vi "CriticalComponents.vi"() -> ()   [LabVIEW 2014]
uses:
  <vilib>/Instr/_visa.llb/VISA Configure Serial Port (Instr).vi
  <vilib>/FieldPoint/Polymorphic Read.llb/FP Read (Float -IO).vi
  <vilib>/FieldPoint/Polymorphic Write.llb/FP Write (Float -IO).vi
  <vilib>/FieldPoint/Polymorphic Write.llb/FP Write (Boolean -IO).vi
  GlobalVariables.vi
panel:
  in  "Tab Control":enum32{"Main", "Email/Text", "Errors", "Misc."}(tab)
  in  "Detector":bool
  in  "Shield":bool
  in  "SC":bool
  out "Pos. Current Readout 2":dbl=1e-05 format="%#.2g"
  out "Neg. Current Readout 2":dbl=1e-05 format="%#.2g"
  out "+ Plate (kV)":dbl
  out "- Plate (kV)":dbl
  out "Current status":bool
  out "Current status 2":bool
  in  "WF Set Point":dbl=0.01 min=0.0 max=10.0 step=0.01 format="%#_3g"
  in  "Auto-Set WF":bool
  in  "Master Voltage control":dbl caption="Set both plate voltages" min=0.0 max=10.0 step=0.01 format="%#_3g"
  in  "stop":bool
  out "Mag. Field (T)":string
  out "Spec Vac":bool
  in  "Spec":bool=TRUE
  out "SC Vac":bool
  in  "SC":bool=TRUE
  out "BL Vac":bool
  in  "BL":bool=TRUE
  in  "Spec turbo\nvalve ctrl":bool
  out "Boolean 9":bool
  in  "Boolean 15":bool
  out "Boolean 8":bool
  in  "BL Ctrl":bool
  out "Boolean 11":bool
  out "Boolean 12":bool
  out "Boolean 13":bool
  in  "Alpha Ctrl":bool
  out "Boolean 10":bool
  in  "Fil on/ 21":bool
  in  "Fil off/ 20":bool
  out "Scat. Chamber":string
  out "Scatt TC (Torr)":string
  in  "BL IG Fil on":bool
  in  "BL IG Fil off":bool
  in  "BL Degas on":bool
  out "Beamline":string
  out "Beamline TC1 (Torr) 2":string
  out "Spectrograph\nVacuum":string
  out "Spectrograph 2 (High Vac)":string
  in  "phone number":string
  in  "Carrier":enum16{"T-Mobile", "AT&T", "Verizon", "Sprint"}(ring)
  in  "On Call":bool
  in  "Write":bool
  in  "Text Body":string
  in  "Text Subject":string="Vacuum Status!"
  in  "Tyler":bool=TRUE
  in  "Michael":bool=TRUE
  in  "Karen":bool=TRUE
  in  "sendbutton":bool
  in  "Tyler Email":bool=TRUE
  in  "Michael Email":bool=TRUE
  in  "Karen Email":bool=TRUE
  in  "Email Message":string caption="Message"
  in  "Email Subject":string caption="Subject"
  in  "Email Send":bool
  out "WF Pos Current":errorcluster caption="error out"
  out "WF Pos Voltage":errorcluster caption="error out"
  out "Spec Ctrl":errorcluster caption="error out"
  out "Spec Close":errorcluster caption="error out"
  out "Spec Open":errorcluster caption="error out"
  out "BL Ctrl 2":errorcluster caption="error out"
  out "BL Close":errorcluster caption="error out"
  out "BL Open":errorcluster caption="error out"
  out "Alpha Ctrl 2":errorcluster caption="error out"
  out "Alpha Close":errorcluster caption="error out"
  out "Alpha Open":errorcluster caption="error out"
  out "WF Neg Current":errorcluster caption="error out"
  out "WF Neg Voltage":errorcluster caption="error out"
  out "BL Cup Error Status":errorcluster caption="error out"
  in  "WF, Comm 34, F":refnum<visa-resource-name>="COM34"
  in  "Spect Vac, Comm 35, A":refnum<visa-resource-name>="COM35"
  in  "BL Vac, Comm 32, G":refnum<visa-resource-name>="COM32"
  out "WF Volt Error":errorcluster caption="error out"
  out "WF Volt Error 2":errorcluster caption="error out"
  out "6600 V1":dbl
  out "6600 V3":dbl
  out "4500 TC1":dbl
  out "4500 IG":dbl
  out "4500 TC2":dbl
  out "4500 TC1 2":dbl
  out "Beamline TC1 (Torr)":string
  out "Spec 2 (high vac) hidden":dbl
  out "x-y":i32
  in  "BL Degas off":bool
  out "Boolean 14":bool
  out "?":bool=TRUE
  out "Vac Indicator":bool=TRUE
  in  "GFM":bool
  in  "Vanilla IC":bool=TRUE
  in  "smtp server":string="smtp.gmail.com"
  in  "show errors 2":bool
  in  "Teslameter Port 5":refnum<visa-resource-name>="COM34"
  # "Overrrides"
  # "Select who receives the email. Green=recieves, Grey =doesn't receive."
  # "Select who receives the text. Green = recieves. Grey = doesn't recieve."
  # "Beam Line IG"
  # "Variable for WF Auto Set"
  # "Scattering Chamber IC"
  # "Not currently working"
  # "For sending emails"
  # "Indicators and Controls not in use."
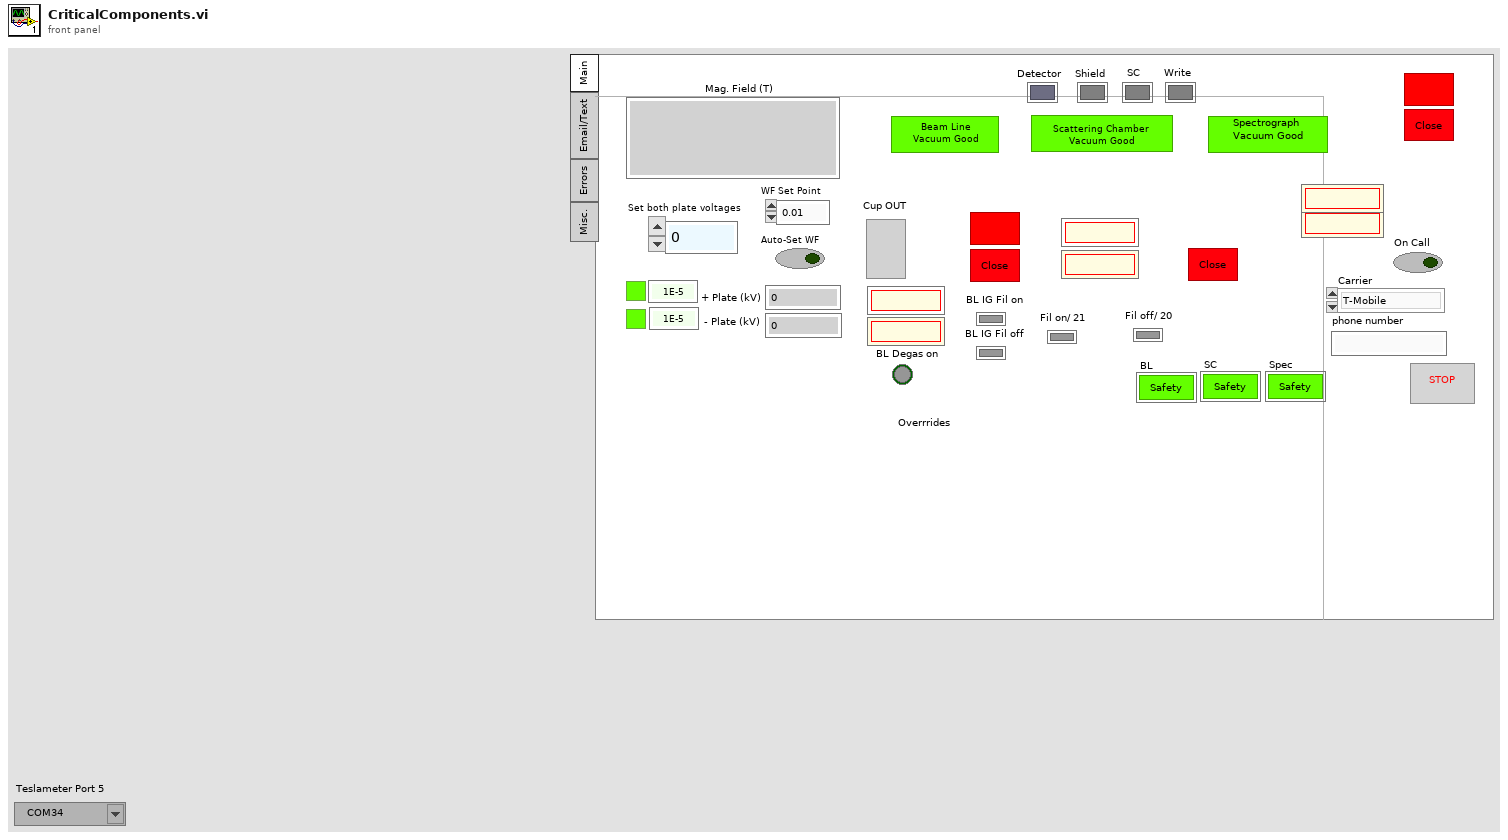
[diagram p1: front panel]
types:
  T1 = enum32{"Invalid", "Standard", "Closed", "Hidden", "Minimized", "Maximized"}
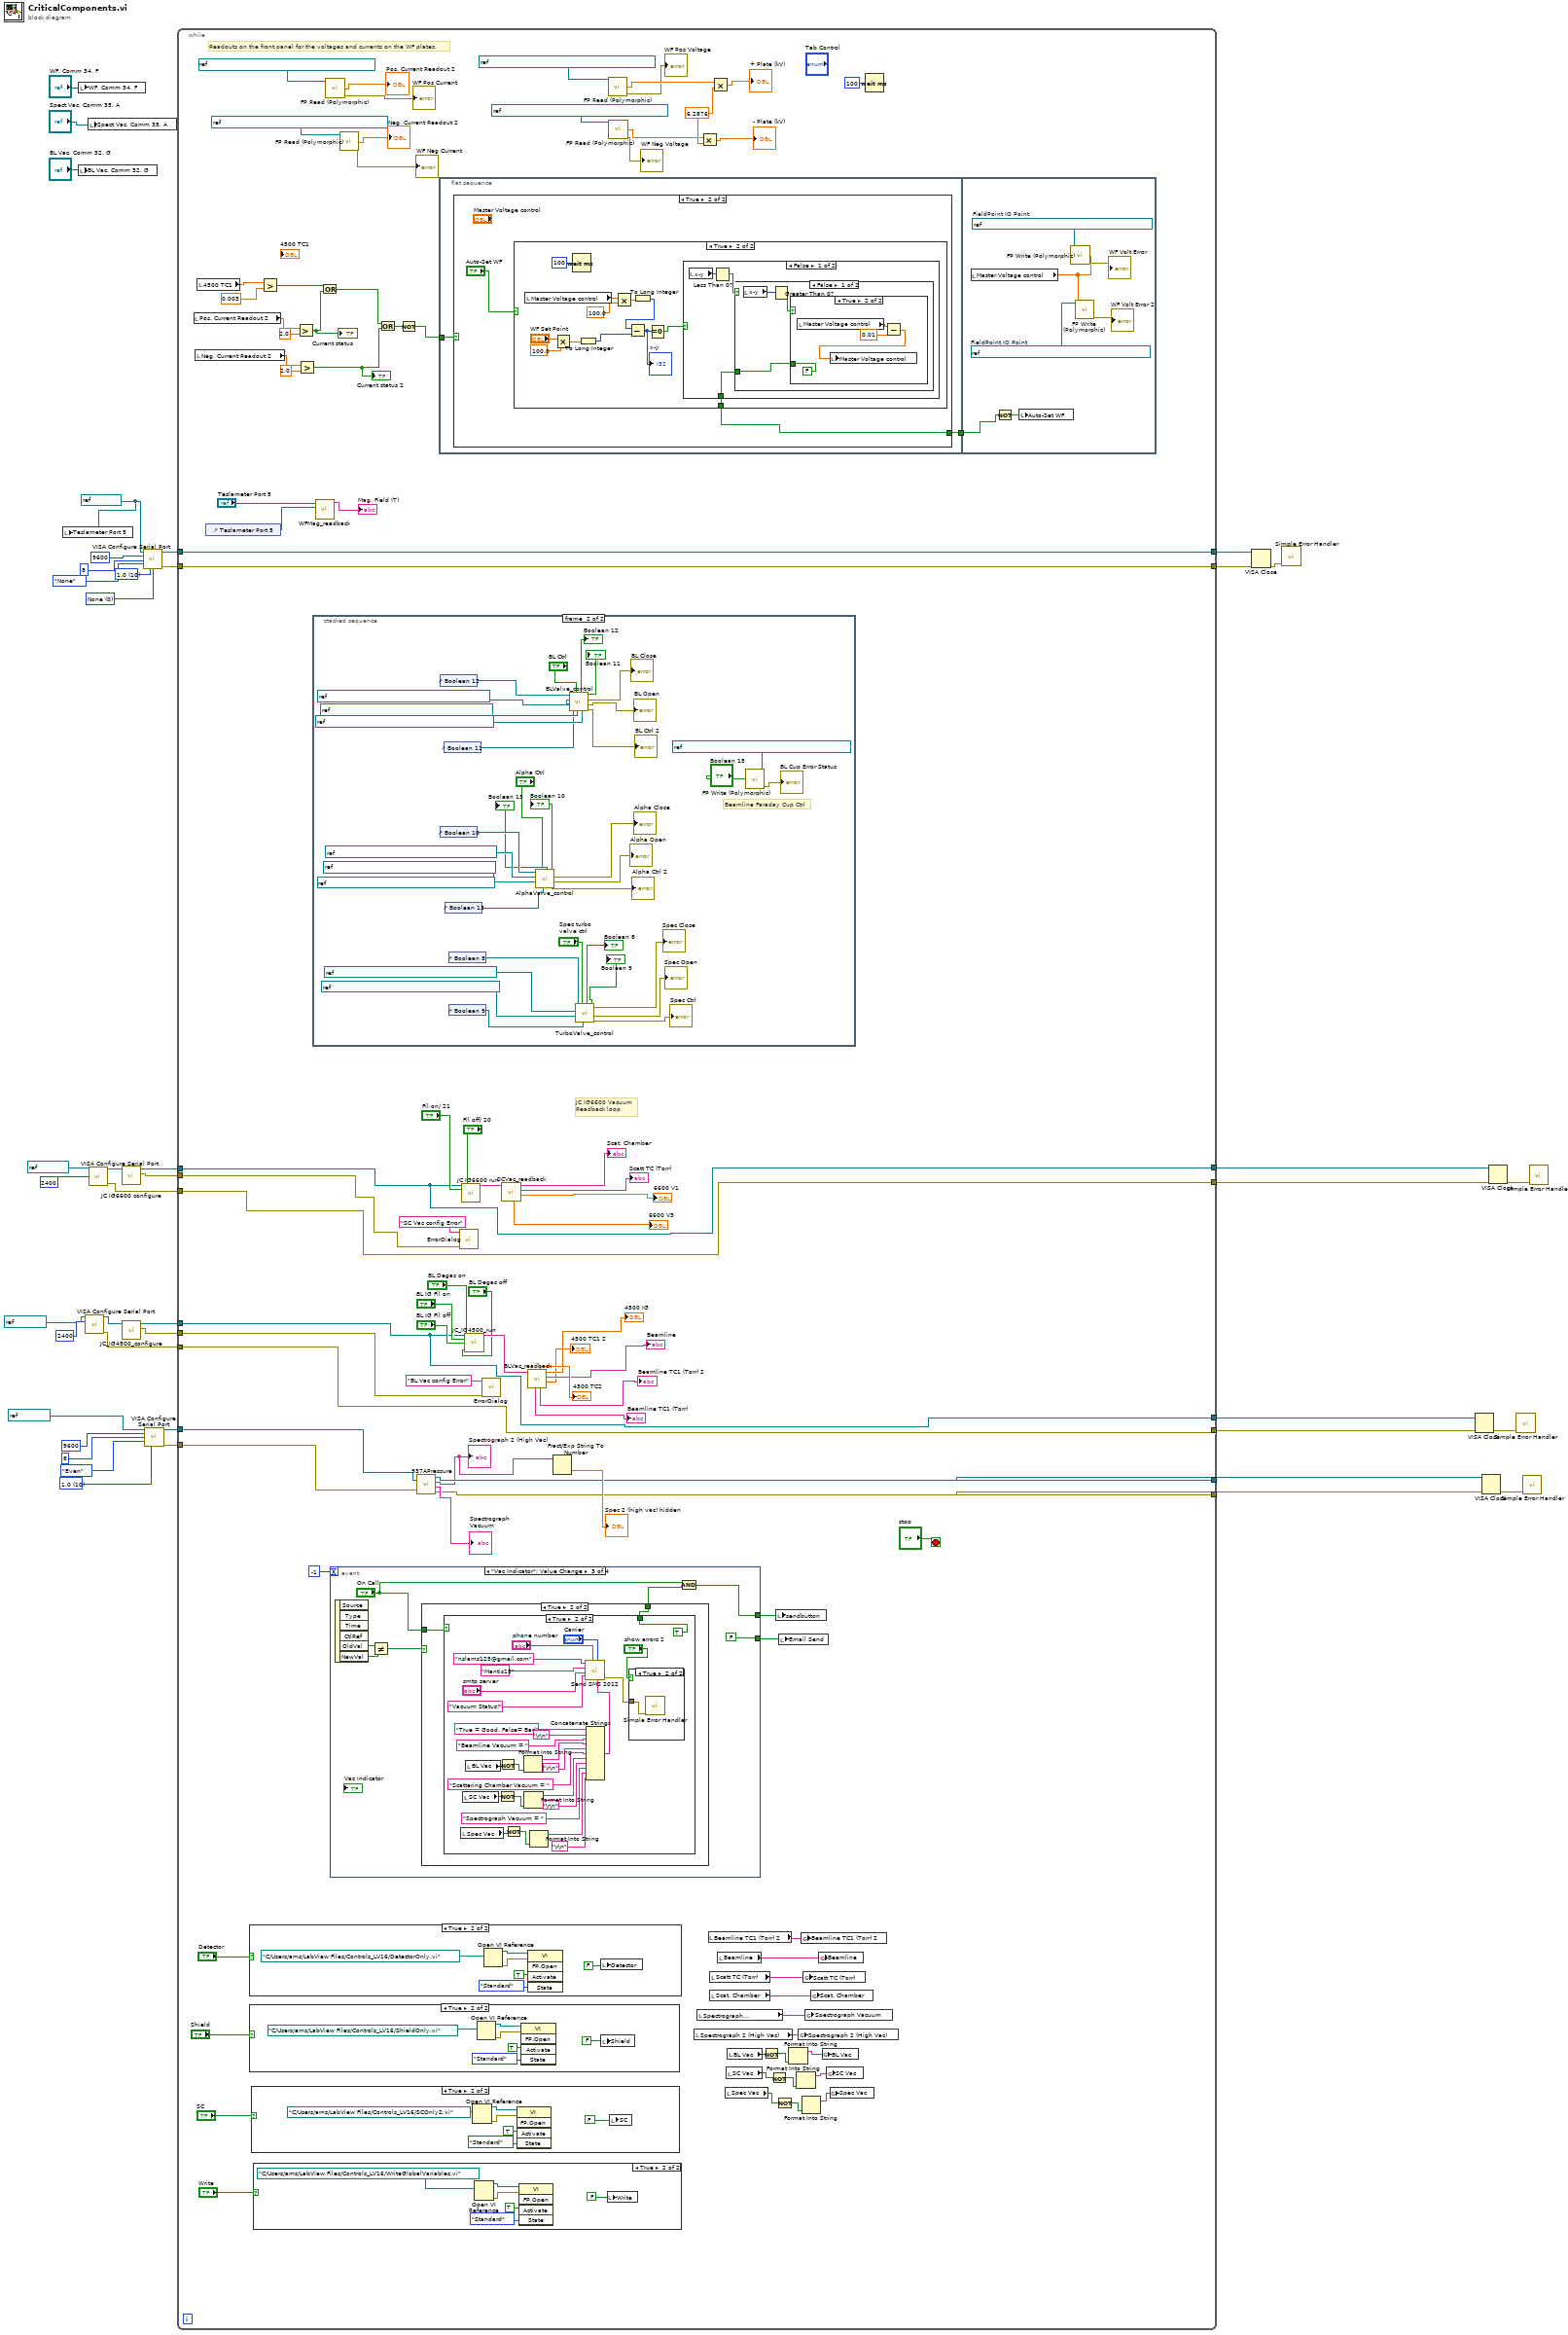
[diagram p0: block diagram]
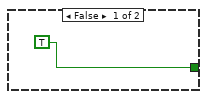
[diagram p2: hidden frame]
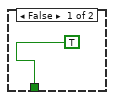
[diagram p3: hidden frame]
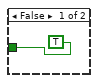
[diagram p4: hidden frame]
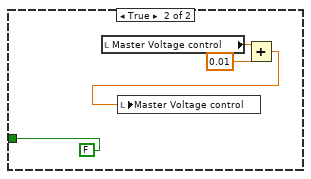
[diagram p5: hidden frame]
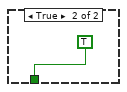
[diagram p6: hidden frame]
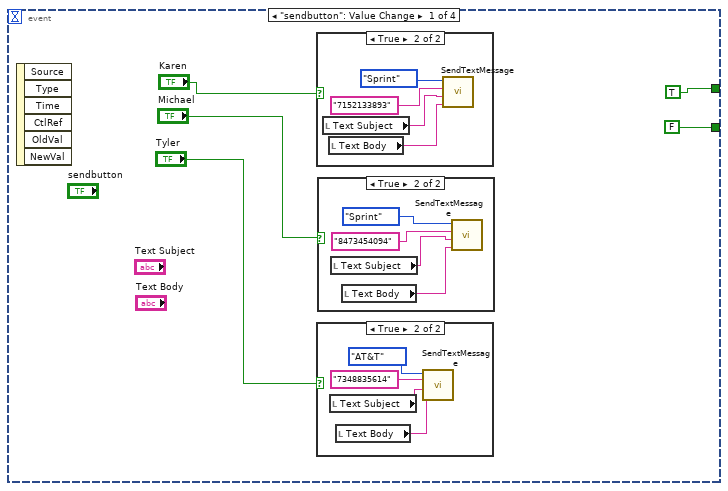
[diagram p11: hidden frame]
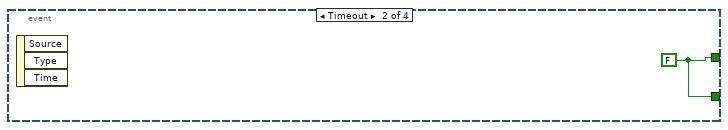
[diagram p15: hidden frame]
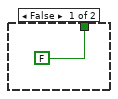
[diagram p16: hidden frame]
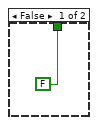
[diagram p17: hidden frame]
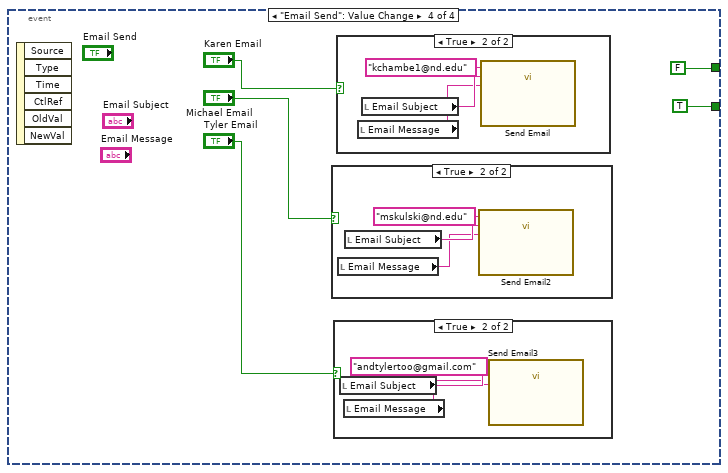
[diagram p19: hidden frame]
diagram:
  w7 = u16 10 items=["1.0"=10, "1.5"=15, "2.0"=20] ("stop bits (10: 1 bit)")
  w34 = refnum<visa-resource-name> "COM34" ("VISA resource name")
  w35 = u16 0 items=["None", "XON/XOFF", "RTS/CTS", "XON/XOFF & RTS/CTS", "DTR/DSR", "XON/XOFF & DTR/DSR"] ("flow control (0:none)")
  w36 = u16 10 items=["1.0"=10, "1.5"=15, "2.0"=20] ("stop bits (10: 1 bit)")
  n1 = local write "Teslameter Port 5"(w34) -> ()
  n2 = local write "BL Vac, Comm 32, G"("BL Vac, Comm 32, G") -> ()
  n3 = local write "WF, Comm 34, F"("WF, Comm 34, F") -> ()
  n4 = call-poly "VISA Configure Serial Port"("VISA resource name"=refnum<visa-resource-name> "COM32" ("VISA IN (Default COM9)"), "baud rate (9600)"=u32 2400) -> ("VISA resource name out"=w13:refnum<visa-resource-name>, "error out"=w8:errorcluster)  [unwired: 12 in]
  n5 = local write "Spect Vac, Comm 35, A"("Spect Vac, Comm 35, A") -> ()
  n6 = call-poly "VISA Configure Serial Port"("VISA resource name"=refnum<visa-resource-name> "COM31" ("VISA IN (Default COM4)"), "baud rate (9600)"=u32 2400) -> ("VISA resource name out"=w19:refnum<visa-resource-name>, "error out"=w15:errorcluster)  [unwired: 12 in]
  n7 = call "JC IG6600 configure.vi"("VISA IN (Default COM4)"=w19) -> ("Error"=w14:errorcluster, "VISA resource name out"=w16:refnum<visa-resource-name>)  [unwired: 9 in]
  n8 = call "JC_IG4500_configure.vi"("VISA IN (Default COM9)"=w13) -> ("Error"=w9:errorcluster, "VISA resource name out"=w10:refnum<visa-resource-name>)  [unwired: 9 in]
  n9 = call-poly "VISA Configure Serial Port"("VISA resource name"=w34, "baud rate (9600)"=u32 9600, "data bits (8)"=u16 8, "parity (0:none)"=enum16{"None", "Odd", "Even", "Mark", "Space"}."None", "stop bits (10: 1 bit)"=w36, "flow control (0:none)"=w35) -> ("VISA resource name out"=w33:refnum<visa-resource-name>, "error out"=w32:errorcluster)  [unwired: 8 in]
  n10 = call-poly "VISA Configure Serial Port"("VISA resource name"=refnum<visa-resource-name> "COM35", "baud rate (9600)"=u32 9600, "data bits (8)"=u16 8, "parity (0:none)"=enum16{"None", "Odd", "Even", "Mark", "Space"}."Even", "stop bits (10: 1 bit)"=w7) -> ("VISA resource name out"=w2:refnum<visa-resource-name>, "error out"=w1:errorcluster)  [unwired: 9 in]
  n11 = while {
    tunnel: w33 -> [w102]
    tunnel: w32 -> [w101]
    tunnel: [w102] -> w30
    tunnel: [w101] -> w31
    tunnel: [w50] -> w26
    tunnel: [w47] -> w28
    tunnel: [w56] -> w24
    tunnel: [w55] -> w23
    tunnel: [w51] -> w21
    tunnel: [w53] -> w20
    tunnel: w16 -> [w56]
    tunnel: w15 -> [w55]
    tunnel: w14 -> [w54]
    tunnel: w10 -> [w53]
    tunnel: w9 -> [w52]
    tunnel: w8 -> [w51]
    tunnel: w2 -> [w46]
    tunnel: w1 -> [w45]
    stop <- "stop" stop-if-true
    w125 = 6.2876
    # "JC IG6600 Vacuum \nReadback loop"
    # "Readouts on the front panel for the voltages and currents on the WF plates."
    n12 = local read "Pos. Current Readout 2"() -> (w116:dbl)
    n13 = local read "Neg. Current Readout 2"() -> (w112:dbl)
    n14 = local read "4500 TC1"() -> (w118:dbl)
    n15 = control-ref of="Teslameter Port 5"() -> (w105:refnum<vi>)
    n16 = case shown="True" "Detector" {
      frame False {
      }
      frame True {
        n17 = Open VI Reference(vi path=path "C:/Users/ams/LabView Files/Controls_LV16/DetectorOnly.vi") -> (vi reference=w192:refnum<vi>, error out=w197:errorcluster)  [unwired: 5 in]
        n18 = invoke class="VI" method="FP.Open"(reference=w192, error in=w197, "Activate"=TRUE ("Activate?"), "State"=T1."Standard") -> ()  [unwired: 1 in, 5 out]
        n19 = local write "Detector"(FALSE) -> ()
      }
    }
    n20 = case shown="True" "Shield" {
      frame False {
      }
      frame True {
        n21 = Open VI Reference(vi path=path "C:/Users/ams/LabView Files/Controls_LV16/ShieldOnly.vi") -> (vi reference=w186:refnum<vi>, error out=w191:errorcluster)  [unwired: 5 in]
        n22 = invoke class="VI" method="FP.Open"(reference=w186, error in=w191, "Activate"=TRUE ("Activate?"), "State"=T1."Standard") -> ()  [unwired: 1 in, 5 out]
        n23 = local write "Shield"(FALSE ("Boolean 2")) -> ()
      }
    }
    n24 = case shown="True" "SC" {
      frame False {
      }
      frame True {
        n25 = Open VI Reference(vi path=path "C:/Users/ams/LabView Files/Controls_LV16/SCOnly2.vi") -> (vi reference=w180:refnum<vi>, error out=w185:errorcluster)  [unwired: 5 in]
        n26 = invoke class="VI" method="FP.Open"(reference=w180, error in=w185, "Activate"=TRUE ("Activate?"), "State"=T1."Standard") -> ()  [unwired: 1 in, 5 out]
        n27 = local write "SC"(FALSE ("Boolean 3")) -> ()
      }
    }
    n28 = case shown="True" "Write" {
      frame False {
      }
      frame True {
        n29 = Open VI Reference(vi path=path "C:/Users/ams/LabView Files/Controls_LV16/WriteGlobalVariables.vi") -> (vi reference=w174:refnum<vi>, error out=w179:errorcluster)  [unwired: 5 in]
        n30 = invoke class="VI" method="FP.Open"(reference=w174, error in=w179, "Activate"=TRUE ("Activate?"), "State"=T1."Standard") -> ()  [unwired: 1 in, 5 out]
        n31 = local write "Write"(FALSE ("Boolean 3")) -> ()
      }
    }
    n32 = Greater?(x=w118, y=0.003) -> (0:w114:bool)
    n33 = Greater?(x=w116, y=2.0) -> (0:w113:bool)
    "Current status" <- w113
    n34 = Greater?(x=w112, y=2.0) -> (0:w108:bool)
    "Current status 2" <- w108
    n35 = stacked-sequence {
      frame #0 {
        # "Spec."
        # "SC"
        # "BL"
        n36 = case shown="True" "Spec" {
          frame False {
          }
          frame True {
            n37 = local read "Spec 2 (high vac) hidden"() -> (w284:dbl)
            n38 = Equal?(x=w284, y=0.0) -> (x = y?=w282:bool)
            n39 = Greater?(x=w284, y=0.0001) -> (0:w281:bool)
            n40 = Or(x=w282, y=w281) -> (x .or. y?=w278:bool)
            "Spec Vac" <- w278
            n41 = case shown="False" "Vanilla IC" {
              tunnel: w278 -> [w291 w294]
              frame False {
                n42 = case shown="True" w291 {
                  selector: w291 -> [_ w293]
                  frame False {
                  }
                  frame True {
                    # "Spec in Safety + Vanilla IC = \nonly Turbo will close."
                    n43 = Not(x=w293) -> (.not. x?=w292:bool)
                    n44 = local write "Spec turbo\nvalve ctrl"(w292) -> ()
                  }
                }
              }
              frame True {
                # "Spec in Saftey + NO Vanilla IC = \nTurbo and Alpha will close."
                n45 = case shown="False" w294 {
                  selector: w294 -> [_ w296]
                  frame False {
                  }
                  frame True {
                    n46 = Not(x=w296) -> (.not. x?=w295:bool)
                    n47 = local write "Alpha Ctrl"(w295) -> ()
                    n48 = local write "Spec turbo\nvalve ctrl"(w295) -> ()
                  }
                }
              }
            }
            n49 = case shown="False" "GFM" {
              tunnel: w278 -> [w287 w288]
              frame False {
                # "Spec in Safety + GFM =\nTurbo will close."
                n50 = Not(x=w287) -> (.not. x?=w286:bool)
                n51 = local write "Spec turbo\nvalve ctrl"(w286) -> ()
              }
              frame True {
                # "Spec in Safety + NON GFM=\nTurbo and Alpha will close."
                n52 = case shown="True" w288 {
                  selector: w288 -> [_ w290]
                  frame False {
                  }
                  frame True {
                    n53 = Not(x=w290) -> (.not. x?=w289:bool)
                    n54 = local write "Spec turbo\nvalve ctrl"(w289) -> ()
                    n55 = local write "Alpha Ctrl"(w289) -> ()
                  }
                }
              }
            }
            "?" <- "Vanilla IC"
            "Boolean 14" <- "GFM"
          }
        }
        n56 = case shown="True" "BL" {
          frame False {
            # "Beamline Override= BL will not close."
            n57 = local read "4500 IG"() -> (w307:dbl)
            n58 = Greater?(x=w307, y=0.0001) -> (0:w305:bool)
            n59 = local write "BL Vac"(w305) -> ()
          }
          frame True {
            n60 = local read "4500 IG"() -> (w310:dbl)
            n61 = Greater?(x=w310, y=0.0001) -> (0:w308:bool)
            "BL Vac" <- w308
            n62 = case shown="False" w308 {
              selector: w308 -> [_ w311]
              frame False {
              }
              frame True {
                n63 = Not(x=w311) -> (.not. x?=w312:bool)
                n64 = local write "BL Ctrl"(w312) -> ()
              }
            }
          }
        }
        n65 = local read "Spec Vac"() -> (w271:bool)
        n66 = local read "BL Vac"() -> (w274:bool)
        n67 = local read "SC Vac"() -> (w273:bool)
        n68 = Or(x=w274, y=w273) -> (x .or. y?=w272:bool)
        n69 = Or(x=w272, y=w271) -> (x .or. y?=w270:bool)
        n70 = Not(x=w270) -> (.not. x?=w269:bool)
        n71 = property on="Vac Indicator" class="Bool (strict)"("Val(Sgnl)"=w269) -> ()  [unwired: 2 in, 2 out]
        n72 = case shown="True" "SC" {
          frame False {
            n73 = local read "6600 V1"() -> (w299:dbl)
            n74 = Greater?(x=w299, y=0.0001) -> (0:w297:bool)
            n75 = local write "SC Vac"(w297) -> ()
          }
          frame True {
            n76 = local read "6600 V1"() -> (w302:dbl)
            n77 = Greater?(x=w302, y=0.0001) -> (0:w300:bool)
            "SC Vac" <- w300
            n78 = case shown="False" w300 {
              selector: w300 -> [_ w304]
              frame False {
              }
              frame True {
                n79 = Not(x=w304) -> (.not. x?=w303:bool)
                n80 = local write "Alpha Ctrl"(w303) -> ()
                n81 = local write "BL Ctrl"(w303) -> ()
              }
            }
          }
        }
      }
      frame #1 {
        # "Beamline Faraday Cup Ctrl"
        n82 = control-ref of="Boolean 12"() -> (w326:refnum<vi>)
        n83 = control-ref of="Boolean 10"() -> (w344:refnum<vi>)
        n84 = control-ref of="Boolean 11"() -> (w332:refnum<vi>)
        n85 = control-ref of="Boolean 13"() -> (w343:refnum<vi>)
        n86 = control-ref of="Boolean 8"() -> (w319:refnum<vi>)
        n87 = control-ref of="Boolean 9"() -> (w318:refnum<vi>)
        n88 = call "AlphaValve_control.vi"("FieldPoint IO Point"=refnum<k21> "FieldPoint\\FP @ COM33\\FP-DIO-550 @2\\Output 1", "reference in"=w343, "OK Button 8"="Alpha Ctrl", "FieldPoint IO Point 2"=refnum<k21> "FieldPoint\\FP @ COM33\\FP-DIO-550 @2\\Input 1" ("FieldPoint IO Point"), "FieldPoint IO Point 3"=refnum<k21> "FieldPoint\\FP @ COM33\\FP-DIO-550 @2\\Input 6" ("FieldPoint IO Point"), "Boolean in"=w344) -> ("error out"=→"Alpha Ctrl 2":errorcluster, "Alpha Open"=→"Alpha Open":errorcluster, "Alpha Close"=→"Alpha Close":errorcluster, "Boolean 10"=→"Boolean 10":bool, "Boolean 13"=→"Boolean 13":bool)  [unwired: 1 in]
        n89 = call "BLValve_control.vi"("FieldPoint IO Point 2"=refnum<k21> "FieldPoint\\FP @ COM33\\FP-DIO-550 @2\\Output 2" ("FieldPoint IO Point"), "FieldPoint IO Point 3"=refnum<k21> "FieldPoint\\FP @ COM33\\FP-DIO-550 @2\\Input 2" ("FieldPoint IO Point"), "OK Button 7"="BL Ctrl", "FieldPoint IO Point"=refnum<k21> "FieldPoint\\FP @ COM33\\FP-DIO-550 @2\\Input 7", "reference in"=w332, "Boolean in"=w326) -> ("error out"=→"BL Ctrl 2":errorcluster, "BL Open"=→"BL Open":errorcluster, "BL Close"=→"BL Close":errorcluster, "Boolean 11"=→"Boolean 11":bool, "Boolean 12"=→"Boolean 12":bool)  [unwired: 1 in]
        n90 = call "TurboValve_control.vi"("Bool Refnum"=w318, "Spec turbo\nvalve ctrl"="Spec turbo\nvalve ctrl", "FieldPoint IO Point"=refnum<k21> "FieldPoint\\FP @ COM33\\FP-DIO-550 @2\\Output 0", "FieldPoint IO Point 2"=refnum<k21> "FieldPoint\\FP @ COM33\\FP-DIO-550 @2\\Input 3" ("FieldPoint IO Point"), "Boolean in"=w319) -> ("error out"=→"Spec Ctrl":errorcluster, "Spec Open"=→"Spec Open":errorcluster, "Spec Close"=→"Spec Close":errorcluster, "Boolean 9"=→"Boolean 9":bool, "Boolean 8"=→"Boolean 8":bool)  [unwired: 2 in]
        n91 = call-poly <vilib>:"FP Write (Polymorphic).vi"("FieldPoint IO Point In"=refnum<k21> "FieldPoint\\FP @ COM33\\FP-DIO-550 @2\\Output 4" ("FieldPoint IO Point"), "value"="Boolean 15") -> ("error out"=→"BL Cup Error Status":errorcluster)  [unwired: 11 in, 2 out]
      }
    }
    n92 = call "WFMag_readback.vi"("reference"=w105, "VISA Refnum in"="Teslameter Port 5") -> ("Mag. Field (T)"=→"Mag. Field (T)":string)  [unwired: 9 in]
    n93 = Or(x=w114, y=w113) -> (x .or. y?=w110:bool)
    n94 = call-poly <vilib>:"FP Read (Polymorphic).vi"("FieldPoint IO Point In"=refnum<k21> "FieldPoint\\FP @ COM33\\FP-AI-112 @1\\Channel 4" ("FieldPoint IO Point")) -> ("value"=→"Pos. Current Readout 2":dbl, "error out"=→"WF Pos Current":errorcluster)  [unwired: 11 in, 2 out]
    n95 = event shown="[2] \"Vac Indicator\": Value Change" {
      selector: _ -> [_ _ _ _]
      dyn-events: _ -> [_ _ _ _]
      timeout: -1 -> [_ _ _ _]
      tunnel: [TRUE w215 w219 FALSE] -> w77
      tunnel: [FALSE w215 FALSE TRUE] -> w79
      event "sendbutton": Value Change {
        n96 = event-data() -> ()  [unwired: 1 in, 6 out]
        n97 = case shown="True" "Karen" {
          frame False {
          }
          frame True {
            n98 = local read "Text Subject"() -> (w212:string)
            n99 = local read "Text Body"() -> (w211:string)
            n100 = call "SendTextMessage.vi"("Body"=w211, "Subject"=w212, "phone number"="7152133893", "Carrier"=enum16{"T-Mobile", "AT&T", "Verizon", "Sprint"}."Sprint") -> ()  [unwired: 8 in]
          }
        }
        n101 = case shown="True" "Tyler" {
          frame False {
          }
          frame True {
            n102 = local read "Text Subject"() -> (w205:string)
            n103 = local read "Text Body"() -> (w204:string)
            n104 = call "SendTextMessage.vi"("Body"=w204, "Subject"=w205, "phone number"="7348835614", "Carrier"=enum16{"T-Mobile", "AT&T", "Verizon", "Sprint"}."AT&T") -> ()  [unwired: 8 in]
          }
        }
        n105 = case shown="True" "Michael" {
          frame False {
          }
          frame True {
            n106 = local read "Text Subject"() -> (w208:string)
            n107 = local read "Text Body"() -> (w207:string)
            n108 = call "SendTextMessage.vi"("Body"=w207, "Subject"=w208, "phone number"="8473454094", "Carrier"=enum16{"T-Mobile", "AT&T", "Verizon", "Sprint"}."Sprint") -> ()  [unwired: 8 in]
          }
        }
      }
      event Timeout {
        w215 = FALSE
        n109 = event-data() -> ()  [unwired: 1 in, 3 out]
      }
      event "Vac Indicator": Value Change {
        n110 = event-data() -> ("OldVal"=w221:bool, "NewVal"=w222:bool)  [unwired: 1 in, 4 out]
        n111 = Not Equal?(x=w221, y=w222) -> (x != y?=w217:bool)
        n112 = case shown="True" w217 {
          tunnel: [FALSE w225] -> w220
          tunnel: "On Call" -> [_ w224]
          frame False {
          }
          frame True {
            n113 = case shown="True" w224 {
              tunnel: [FALSE TRUE] -> w225
              frame False {
              }
              frame True {
                n114 = local read "Spec Vac"() -> (w233:bool)
                n115 = local read "SC Vac"() -> (w239:bool)
                n116 = local read "BL Vac"() -> (w244:bool)
                n117 = Not(x=w239) -> (.not. x?=w238:bool)
                n118 = Not(x=w244) -> (.not. x?=w243:bool)
                n119 = Not(x=w233) -> (.not. x?=w234:bool)
                n120 = Format Into String(w243) -> (resulting string=w242:string)  [unwired: 3 in, 1 out]
                n121 = Format Into String(w238) -> (resulting string=w237:string)  [unwired: 3 in, 1 out]
                n122 = Format Into String(w234) -> (resulting string=w232:string)  [unwired: 3 in, 1 out]
                n123 = Concatenate Strings("True = Good, False= Bad" ("string"), "\r\n", "Beamline Vacuum = ", w242, "\r\n", "Scattering Chamber Vacuum = ", w237, "\r\n", "Spectrograph Vacuum = ", w232, "\r\n") -> (w230:string)
                n124 = call "Send SMS 2012.vi"("Body"=w230, "Carrier"="Carrier", "Subject"="Vacuum Status!", "phone number"="phone number", "smtp server"="smtp server", "password"="Mantis15", "email username"="nslams125@gmail.com") -> ("Error Out"=w228:errorcluster)  [unwired: 4 in]
                n125 = case shown="True" "show errors 2" {
                  tunnel: w228 -> [_ w254]
                  frame False {
                  }
                  frame True {
                    n126 = call <vilib>:"Simple Error Handler.vi"("error in (no error)"=w254) -> ()  [unwired: 4 in, 5 out]
                  }
                }
              }
            }
          }
        }
        n127 = And(x="On Call", y=w220) -> (x .and. y?=w219:bool)
      }
      event "Email Send": Value Change {
        n128 = event-data() -> ()  [unwired: 1 in, 6 out]
        n129 = case shown="True" "Michael Email" {
          frame False {
          }
          frame True {
            n130 = local read "Email Message"() -> (w263:string)
            n131 = local read "Email Subject"() -> (w264:string)
            n132 = call "Send Email2"("Message"=w263, "Subject"=w264, "Recipients"="mskulski@nd.edu") -> ()  [unwired: 8 in, 1 out]
          }
        }
        n133 = case shown="True" "Tyler Email" {
          frame False {
          }
          frame True {
            n134 = local read "Email Subject"() -> (w261:string)
            n135 = local read "Email Message"() -> (w260:string)
            n136 = call "Send Email3"("Message"=w260, "Subject"=w261, "Recipients"="andtylertoo@gmail.com") -> ()  [unwired: 8 in, 1 out]
          }
        }
        n137 = case shown="True" "Karen Email" {
          frame False {
          }
          frame True {
            n138 = local read "Email Message"() -> (w266:string)
            n139 = local read "Email Subject"() -> (w267:string)
            n140 = call "Send Email"("Message"=w266, "Subject"=w267, "Recipients"="kchambe1@nd.edu") -> ()  [unwired: 8 in, 1 out]
          }
        }
      }
    }
    n141 = call-poly <vilib>:"FP Read (Polymorphic).vi"("FieldPoint IO Point In"=refnum<k21> "FieldPoint\\FP @ COM33\\FP-AI-112 @1\\Channel 5" ("FieldPoint IO Point")) -> ("value"=→"Neg. Current Readout 2":dbl, "error out"=→"WF Neg Current":errorcluster)  [unwired: 11 in, 2 out]
    n142 = Or(x=w110, y=w108) -> (x .or. y?=w109:bool)
    n143 = Not(x=w109) -> (.not. x?=w107:bool)
    n144 = call "937APressure.vi"("VISA resource name"=w46, "error in (no error)"=w45) -> ("VISA resource name out"=w50:refnum<visa-resource-name>, "Hi Spect"=w49:string, "Lo Spect"=→"Spectrograph\nVacuum":string, "error out"=w47:errorcluster)
    "Spectrograph 2 (High Vac)" <- w49
    n145 = flat-sequence {
      tunnel: w107 -> [w134]
      tunnel: [w133] -> w43
      tunnel: w43 -> [w167]
      frame #0 {
        n146 = case shown="True" w134 {
          tunnel: [TRUE w136] -> w133
          frame False {
          }
          frame True {
            n147 = case shown="True" "Auto-Set WF" {
              tunnel: [TRUE w140] -> w136
              frame False {
              }
              frame True {
                n148 = local read "Master Voltage control"() -> (w150:dbl)
                n149 = Multiply(x="WF Set Point", y=100.0) -> (x*y=w145:dbl)
                n150 = Wait (ms)(milliseconds to wait=u32 100) -> ()  [unwired: 1 out]
                n151 = To Long Integer(number=w145) -> (32bit integer=w143:i32)
                n152 = Multiply(x=w150, y=100.0) -> (x*y=w148:dbl)
                n153 = To Long Integer(number=w148) -> (32bit integer=w144:i32)
                n154 = Subtract(x=w144, y=w143) -> (x-y=w142:i32)
                "x-y" <- w142
                n155 = Equal To 0?(x=w142) -> (x = 0?=w141:bool)
                n156 = case shown="False" w141 {
                  tunnel: [w151 TRUE] -> w140
                  frame False {
                    n157 = local read "x-y"() -> (w153:i32)
                    n158 = Less Than 0?(x=w153) -> (x < 0?=w152:bool)
                    n159 = case shown="False" w152 {
                      tunnel: [w154 FALSE] -> w151
                      frame False {
                        n160 = local read "x-y"() -> (w156:i32)
                        n161 = Greater Than 0?(x=w156) -> (x > 0?=w155:bool)
                        n162 = case shown="True" w155 {
                          tunnel: [TRUE FALSE] -> w154
                          frame False {
                          }
                          frame True {
                            n163 = local read "Master Voltage control"() -> (w161:dbl)
                            n164 = Subtract(x=w161, y=0.01) -> (x-y=w159:dbl)
                            n165 = local write "Master Voltage control"(w159) -> ()
                          }
                        }
                      }
                      frame True {
                        n166 = local read "Master Voltage control"() -> (w164:dbl)
                        n167 = Add(x=w164, y=0.01) -> (x+y=w163:dbl)
                        n168 = local write "Master Voltage control"(w163) -> ()
                      }
                    }
                  }
                  frame True {
                  }
                }
              }
            }
          }
        }
      }
      frame #1 {
        w173 = refnum<k21> "FieldPoint\\FP @ COM33\\FP-AO-210 @4\\Channel 4"  # FieldPoint IO Point
        w169 = refnum<k21> "FieldPoint\\FP @ COM33\\FP-AO-210 @4\\Channel 3"  # FieldPoint IO Point
        n169 = local read "Master Voltage control"() -> (w170:dbl)
        n170 = Not(x=w167) -> (.not. x?=w168:bool)
        n171 = local write "Auto-Set WF"(w168) -> ()
        n172 = call-poly <vilib>:"FP Write (Polymorphic).vi"("FieldPoint IO Point In"=w169, "value"=w170) -> ("error out"=→"WF Volt Error":errorcluster)  [unwired: 11 in, 2 out]
        n173 = call-poly <vilib>:"FP Write (Polymorphic).vi"("FieldPoint IO Point In"=w173, "value"=w170) -> ("error out"=→"WF Volt Error 2":errorcluster)  [unwired: 11 in, 2 out]
      }
    }
    n174 = call "ErrorDialog.vi"("error in (no error)"=w54, "message"="SC Vac config Error") -> ()  [unwired: 10 in]
    n175 = call "JC IG6600 run.vi"("VISA IN"=w56, "Fil on"="Fil on/ 21", "Fil off"="Fil off/ 20") -> ("Readback array"=w100:string[])  [unwired: 11 in, 1 out]
    n176 = call "JC_IG4500_run.vi"("VISA IN"=w53, "Fil on"="BL IG Fil on", "Fil off"="BL IG Fil off", "Degas on"="BL Degas on", "Degas off"="BL Degas off") -> ("Readback array"=w92:string[])  [unwired: 9 in, 1 out]
    n177 = call "ErrorDialog.vi"("error in (no error)"=w52, "message"="BL Vac config Error") -> ()  [unwired: 10 in]
    n178 = call "SCVac_readback.vi"("Readback array"=w100) -> ("6600 V1"=→"6600 V1":dbl, "Scatt TC (Torr)"=→"Scatt TC (Torr)":string, "Scat. Chamber"=→"Scat. Chamber":string, "6600 V3"=→"6600 V3":dbl)  [unwired: 7 in]
    n179 = call "BLVac_readback.vi"("Readback array"=w92) -> ("4500 TC1 2"=→"4500 TC1 2":dbl, "Beamline"=→"Beamline":string, "4500 IG"=→"4500 IG":dbl, "Beamline TC1 (Torr) 2"=→"Beamline TC1 (Torr) 2":string, "4500 TC2"=→"4500 TC2":dbl, "Beamline TC1 (Torr)"=→"Beamline TC1 (Torr)":string)  [unwired: 5 in]
    n180 = Fract/Exp String To Number(string=w49) -> (number=→"Spec 2 (high vac) hidden":dbl)  [unwired: 3 in, 1 out]
    n181 = call-poly <vilib>:"FP Read (Polymorphic).vi"("FieldPoint IO Point In"=refnum<k21> "FieldPoint\\FP @ COM33\\FP-AI-112 @1\\Channel 6" ("FieldPoint IO Point")) -> ("value"=w123:dbl, "error out"=→"WF Pos Voltage":errorcluster)  [unwired: 11 in, 2 out]
    n182 = call-poly <vilib>:"FP Read (Polymorphic).vi"("FieldPoint IO Point In"=refnum<k21> "FieldPoint\\FP @ COM33\\FP-AI-112 @1\\Channel 7" ("FieldPoint IO Point")) -> ("value"=w124:dbl, "error out"=→"WF Neg Voltage":errorcluster)  [unwired: 11 in, 2 out]
    n183 = local read "Spectrograph 2 (High Vac)"() -> (w67:string)
    n184 = local read "Spectrograph\nVacuum"() -> (w68:string)
    n185 = Multiply(x=w124, y=w125) -> (x*y=→"- Plate (kV)":dbl)
    n186 = local read "Beamline TC1 (Torr) 2"() -> (w72:string)
    n187 = local read "Scatt TC (Torr)"() -> (w70:string)
    n188 = local read "Scat. Chamber"() -> (w69:string)
    n189 = Multiply(x=w123, y=w125) -> (x*y=→"+ Plate (kV)":dbl)
    n190 = local read "Beamline"() -> (w71:string)
    n191 = local read "Spec Vac"() -> (w61:bool)
    n192 = local read "SC Vac"() -> (w62:bool)
    n193 = local read "BL Vac"() -> (w63:bool)
    n194 = Not(x=w63) -> (.not. x?=w66:bool)
    n195 = Not(x=w62) -> (.not. x?=w65:bool)
    n196 = Not(x=w61) -> (.not. x?=w64:bool)
    n197 = local write "sendbutton"(w77) -> ()
    n198 = local write "Email Send"(w79) -> ()
    n199 = Format Into String(w66) -> (resulting string=w60:string)  [unwired: 3 in, 1 out]
    n200 = Format Into String(w65) -> (resulting string=w59:string)  [unwired: 3 in, 1 out]
    n201 = global write "GlobalVariables.vi" "Spectrograph 2 (High Vac)"(w67) -> ()
    n202 = global write "GlobalVariables.vi" "Beamline TC1 (Torr) 2"(w72) -> ()
    n203 = Format Into String(w64) -> (resulting string=w58:string)  [unwired: 3 in, 1 out]
    n204 = global write "GlobalVariables.vi" "Scatt TC (Torr)"(w70) -> ()
    n205 = global write "GlobalVariables.vi" "Spectrograph Vacuum"(w68) -> ()
    n206 = global write "GlobalVariables.vi" "Scat. Chamber"(w69) -> ()
    n207 = global write "GlobalVariables.vi" "Beamline"(w71) -> ()
    n208 = global write "GlobalVariables.vi" "BL Vac"(w60) -> ()
    n209 = global write "GlobalVariables.vi" "SC Vac"(w59) -> ()
    n210 = global write "GlobalVariables.vi" "Spec Vac"(w58) -> ()
    n211 = Wait (ms)(milliseconds to wait=u32 100) -> ()  [unwired: 1 out]
  }
  n212 = VISA Close(VISA resource name=w30, error in (no error)=w31) -> (error out=w29:errorcluster)
  n213 = call <vilib>:"Simple Error Handler.vi"("error in (no error)"=w29) -> ()  [unwired: 4 in, 5 out]
  n214 = VISA Close(VISA resource name=w20, error in (no error)=w21) -> (error out=w22:errorcluster)
  n215 = VISA Close(VISA resource name=w26, error in (no error)=w28) -> (error out=w27:errorcluster)
  n216 = VISA Close(VISA resource name=w24, error in (no error)=w23) -> (error out=w25:errorcluster)
  n217 = call <vilib>:"Simple Error Handler.vi"("error in (no error)"=w22) -> ()  [unwired: 4 in, 5 out]
  n218 = call <vilib>:"Simple Error Handler.vi"("error in (no error)"=w27) -> ()  [unwired: 4 in, 5 out]
  n219 = call <vilib>:"Simple Error Handler.vi"("error in (no error)"=w25) -> ()  [unwired: 4 in, 5 out]
